vi "Verify Parameterized.vi"(5 "Label":string, 7 "Approval Tests.lvlib:Options.lvclass":refnum<class "Options.lvclass">, 8 "error in":errorcluster, 9 "Set of ctl label -> value var":set{map{string, variant}}(c389), 10 "VI in":refnum<vi>) -> (0 "error out":errorcluster, 1 "Failure Message":string, 2 "Passed?":bool)   [LabVIEW 2020, in "Approval Tests.lvlib"]
doc: "You pass in a reference to the function you want to test. You also pass in a set of maps. Each map maps each control label to a variant value (You must use the \"to Variant\" primitive or you'll get a broken run arrow due to the type mismatch). The control must be connected to the connector pane. Ideally you would have the same number of elements in your map as controls connected to the connector pane. If you don't specify a value for a control, it just stays whatever the default is set at. The underlying code will cycle through the set and for each map, will set the control values appropriately and then run the vi and capture any indicators connected to the connector pane. The control and corresponding indicator values are all stored in the approved file."
uses:
  Approval Tests.lvlib
  Options/Options.lvclass
  3c7c7814-4b82-40b9-8668-651602b49377.vi
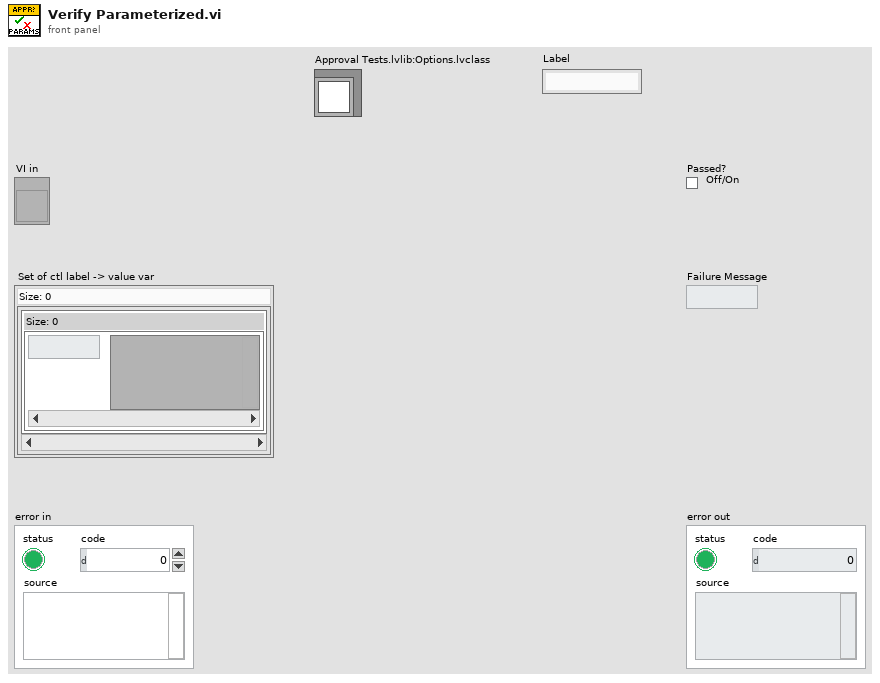
[diagram p1: front panel]
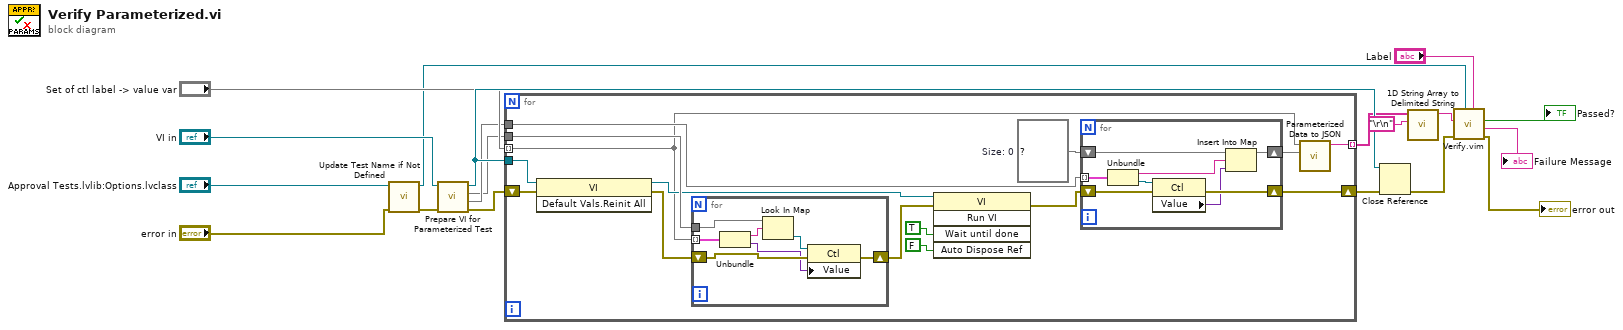
[diagram p0: block diagram]
diagram:
  n1 = call "Update Test Name if Not Defined.vi"("error in"="error in", "Options in"="Approval Tests.lvlib:Options.lvclass") -> ("error out"=w16:errorcluster, "Options out"=w5:refnum<class "Options.lvclass">)  [unwired: 8 in]
  n2 = call "Prepare VI for Parameterized Test.vi"("error in"=w16, "VI in"="VI in") -> ("error out"=w18:errorcluster, "Indicators"=w12:map{string, refnum<vi>}, "Controls"=w11:map{string, refnum<vi>}, "VI out"=w15:refnum<vi>)  [unwired: 6 in]
  n3 = for {
    tunnel: w11 -> [w27]
    tunnel: w12 -> [w26]
    tunnel: w15 -> [w25]
    tunnel: [w22] -> w10 mode=indexing
    tunnel: "Set of ctl label -> value var" -> [w23] mode=indexing
    shift-right: [w30] -> w19
    shift-left: w18 -> [w31]
    w21 = map{string, variant} {}  # Size: 0
    n4 = invoke on="Invoke Node" class="VI" method="Default Vals.Reinit All"(reference=w25, error in=w31) -> (reference out=w24:refnum<vi>, error out=w33:errorcluster)  [unwired: 1 in, 1 out]
    n5 = for {
      tunnel: w27 -> [w47]
      tunnel: w23 -> [w46] mode=indexing
      shift-right: [w49] -> w34
      shift-left: w33 -> [w48]
      n6 = Unbundle(w46) -> ("key"=w45:string, "Variant"=w43:variant)
      n7 = Look In Map(map=w47, key=w45) -> (value=w44:refnum<vi>)  [unwired: 1 in, 1 out]
      n8 = property on="Property Node" class="Ctl"(reference=w44, error in=w48, "Value"=w43) -> (error out=w49:errorcluster)  [unwired: 1 out]
    }
    n9 = invoke on="Invoke Node" class="VI" method="Run VI"(reference=w24, error in=w34, "Wait until done"=TRUE ("Wait Until Done"), "Auto Dispose Ref"=FALSE ("Auto Dispose Reference")) -> (error out=w32:errorcluster)  [unwired: 1 in, 4 out]
    n10 = for {
      tunnel: w26 -> [w40] mode=indexing
      shift-right: [w41] -> w30
      shift-left: w32 -> [w42]
      shift-right: [w36] -> w20
      shift-left: w21 -> [w35]
      n11 = Unbundle(w40) -> (w38:string, "reference"=w39:refnum<vi>)
      n12 = property on="Property Node" class="Ctl"(reference=w39, error in=w42) -> (error out=w41:errorcluster, "Value"=w37:variant)  [unwired: 1 out]
      n13 = Insert Into Map(map in=w35, key=w38, value=w37) -> (map out=w36:map{string, variant})  [unwired: 2 out]
    }
    n14 = call "Parameterized Data to JSON.vi"("Outputs"=w20, "Inputs"=w23) -> ("<JSON>"=w22:string)  [unwired: 9 in]
  }
  n15 = Close Reference(reference=w15, error in (no error)=w19) -> (error out=w7:errorcluster)
  n16 = call <vilib>:"1D String Array to Delimited String.vi"("delimiter"="\r\n", "string array"=w10) -> ("delimited string"=w6:string)  [unwired: 9 in]
  n17 = call "Verify.vim"("Label"="Label", "Options"=w5, "error in"=w7, "Anything"=w6) -> ("error out"=→"error out":errorcluster, "Failure Message"=→"Failure Message":string, "Passed?"=→"Passed?":bool)  [unwired: 5 in]
